vi "Unflatten Value.vi"(8 "error in (no error)":errorcluster, 10 "Value":string, 11 "Boolean in":refnum<class "Boolean.lvclass">) -> (0 "error out":errorcluster, 3 "Boolean out":refnum<class "Boolean.lvclass">)   [LabVIEW 2020, in "Boolean.lvclass"]
uses:
  <vilib>/gpm_packages/@cs/data-type-serializer/source/Boolean/Boolean.lvclass
  <vilib>/gpm_packages/@cs/data-type-serializer/source/Boolean/Boolean.lvclass/Boolean.ctl
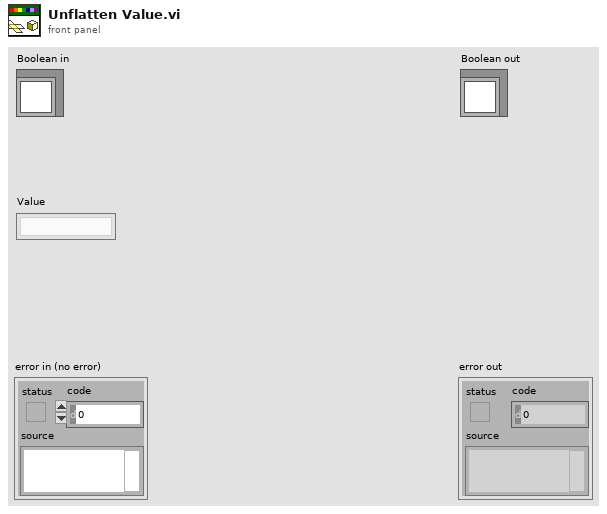
[diagram p1: front panel]
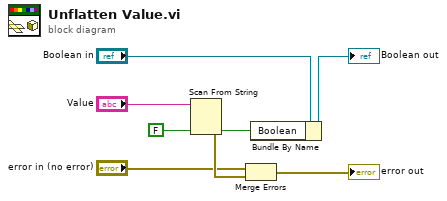
[diagram p0: block diagram]
diagram:
  n1 = Scan From String(input string="Value", default 1=FALSE) -> (error out=w6:errorcluster, output 1=w5:bool)  [unwired: 3 in, 2 out]
  n2 = Merge Errors("error in (no error)", w6) -> (→"error out":errorcluster)
  n3 = Bundle By Name(cluster="Boolean in", "Boolean"=w5) -> (→"Boolean out":refnum<class "Boolean.lvclass">)
